vi "Write configuration.vi"(8 "error in":errorcluster, 10 "configuration":refnum<class "NISE_CEF_serializable configuration.lvclass">, 11 "My System in":refnum<class "My System.lvclass">) -> (0 "error out":errorcluster, 3 "My System out":refnum<class "My System.lvclass">)   [LabVIEW 2014, in "My System.lvclass"]
uses:
  My System.lvclass
  <vilib>/NI/Configuration Framework/serializable configuration/NISE_CEF_serializable configuration.lvclass
  My System Configuration/My System Configuration.lvclass
  My System.lvclass/My System.ctl
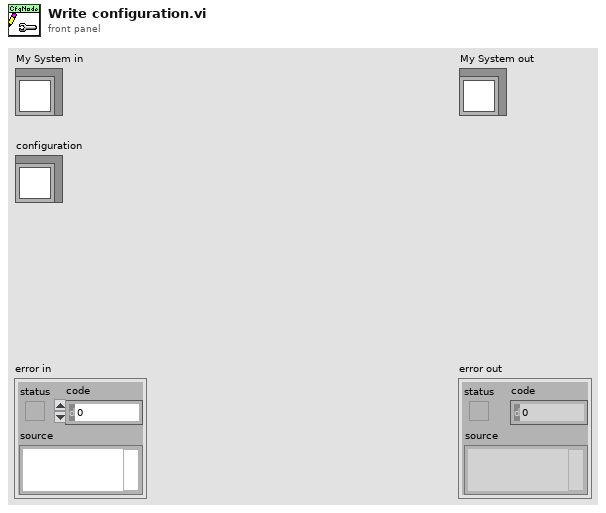
[diagram p1: front panel]
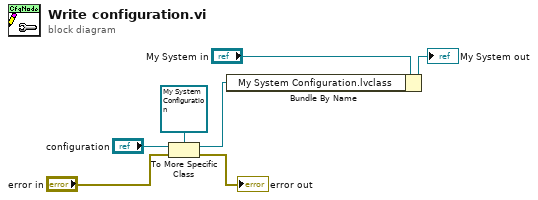
[diagram p0: block diagram]
diagram:
  n1 = To More Specific Class(target class=refnum<class "My System Configuration.lvclass"> refnum ("My System Configuration.lvclass"), reference="configuration", error in="error in") -> (specific class reference=w1:refnum<class "My System Configuration.lvclass">, error out=→"error out":errorcluster)
  n2 = Bundle By Name(cluster="My System in", "My System Configuration.lvclass"=w1) -> (→"My System out":refnum<class "My System.lvclass">)
